vi "nth Derivative of Rational Polynomial.vi"   [LabVIEW 2017, in "NI_AALPro.lvlib"]
doc: "Calculates the nth order derivative of a rational polynomial. The data types you wire to the <B>P(x)</B> and <B>Q(x)</B> inputs determine the polymorphic instance to use."
uses:
  NI_AALPro.lvlib
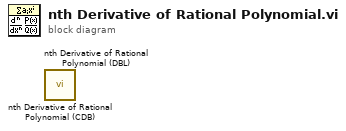
[diagram p0: block diagram]
diagram:
  n1 = call "nth Derivative of Rational Polynomial (CDB).vi"() -> ()  [unwired: 9 in, 3 out]
  n2 = call "nth Derivative of Rational Polynomial (DBL).vi"() -> ()  [unwired: 9 in, 3 out]
